vi "udp LA send convert.vi"() -> ()   [LabVIEW 2017]
uses:
  global variable.vi
panel:
  in  "정지":bool
  out "x*y":dbl
  out "x/y":dbl
  out "숫자":i32
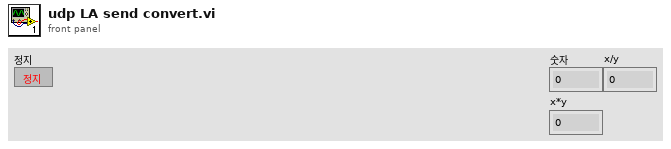
[diagram p1: front panel]
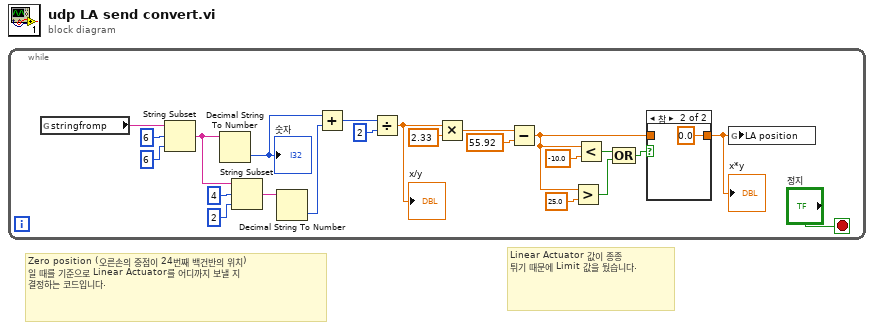
[diagram p0: block diagram]
diagram:
  # "Linear Actuator 값이 종종\n튀기 때문에 Limit 값을 뒀습니다."
  # "Zero position (오른손의 중점이 24번째 백건반의 위치)\n일 때를 기준으로 Linear Actuator를 어디까지 보낼 지\n결정하는 코드입니다."
  n1 = while {
    stop <- "정지" stop-if-true
    n2 = global read "global variable.vi" "stringfromp"() -> (w11:string)
    n3 = String Subset(string=w11, offset (0)=6 ("오프셋(0)"), length (rest)=6 ("길이(나머지)")) -> (substring=w19:string)
    n4 = Decimal String To Number(string=w19) -> (number=w18:i32)  [unwired: 2 in, 1 out]
    "숫자" <- w18
    n5 = String Subset(string=w19, offset (0)=4 ("오프셋(0)"), length (rest)=2 ("길이(나머지)")) -> (substring=w17:string)
    n6 = Decimal String To Number(string=w17) -> (number=w16:i32)  [unwired: 2 in, 1 out]
    n7 = Add(x=w18, y=w16) -> (x+y=w15:i32)
    n8 = Divide(x=w15, y=2) -> (x/y=w13:dbl)
    "x/y" <- w13
    n9 = Multiply(x=w13, y=2.33) -> (x*y=w10:dbl)
    n10 = Subtract(x=w10, y=55.92) -> (x-y=w1:dbl)
    n11 = Greater?(x=w1, y=25.0) -> (0:w5:bool)
    n12 = Less?(x=w1, y=-10.0) -> (x < y?=w7:bool)
    n13 = Compound Arithmetic op=OR ("복합 연산")(w7, w5) -> (w3:bool)
    n14 = case shown="참" w3 {
      tunnel: [w24 0.0] -> w2
      tunnel: w1 -> [w24 _]
      frame False {
      }
      frame True {
      }
    }
    "x*y" <- w2
    n15 = global write "global variable.vi" "LA position"(w2) -> ()
  }
